vi "setPolarity.vi"(0 "SingleAxisController in":refnum<class "_SingleAxisController.lvclass">, 2 "polarity_items (in)":T2[](array[typedef]), 3 "axis (in) - nc-this is only applicable for multi-axis applications":T1, 5 "error in (no error)":errorcluster) -> (14 "SingleAxisController out":refnum<class "_SingleAxisController.lvclass">, 17 "success?":bool, 18 "response":string, 19 "error out":errorcluster)   [LabVIEW 2020, in "classes.lvlib" / "_SingleAxisController.lvclass"]
doc: "Produced By:\n\n<B>Kod Integrations, LLC</B>\n4835 Marianne Drive\nMount Airy, MD 21771\nhttp://www.kodintegrations.com\nemail: info@kodintegrations.com\nphone: (240) 687-1288"
uses:
  _SingleAxisController.lvclass
  C:/GEECS/Developers Version/source/Device Drivers/Newmark-NSC-A/Arcus Driver 3.0.0/ArcusUsbComm/classes/Controller/_Controller.lvclass
  common/controls/polarity_item.ctl
  common/controls/polarity.ctl
  common/controls/axis.ctl
  common/controls/simple_actions.ctl
  libraries/common.lvlib
  Controller/_Controller.lvclass
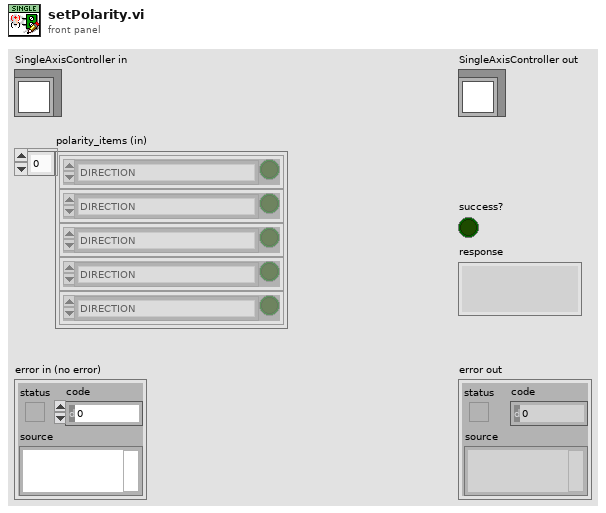
[diagram p1: front panel]
types:
  T1 = typedef "common.lvlib/axis.ctl" = enum16{"X", "Y", "Z", "U"}
  T2 = typedef "common.lvlib/polarity_item.ctl" = cluster{"item":T3, "status":bool}
  T3 = typedef "common.lvlib/polarity.ctl" = enum16{"DIRECTION", "LIMIT", "HOME", "DIG_OUT", "DIG_IN", "ENABLE_OUT", "JUMP_ERR", "LATCH", "Z-CHAN_INDEX", "ENCODER_DECODING:1X", "ENCODER_DECODING:2X", "ENCODER_DECODING:4X", "ALARM", "STANDALONE_ERR", "-", "<reserved/nc>"}
  T4 = typedef "common.lvlib/simple_actions.ctl" = enum16{"from_value", "to_value"}
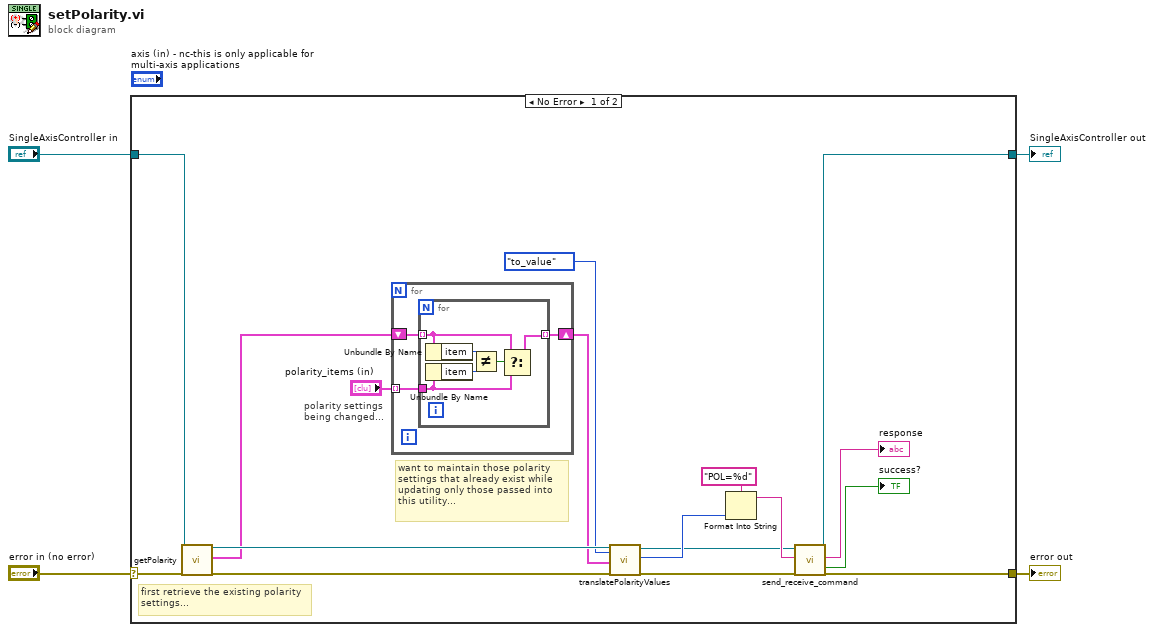
[diagram p0: block diagram]
diagram:
  n1 = case shown="No Error" "error in (no error)" {
    selector: "error in (no error)" -> [w8 w32]
    tunnel: [w7 w32] -> w3
    tunnel: [w5 w31] -> w1
    tunnel: "SingleAxisController in" -> [w6 w31]
    frame No Error {
      # "want to maintain those polarity\nsettings that already exist while\nupdating only those passed into\nthis utility..."
      # "first retrieve the existing polarity\nsettings..."
      # "polarity settings\nbeing changed..."
      n2 = call-dynamic "getPolarity.vi"("reference (in)"=w6, "error in (no error)"=w8) -> ("reference (out)"=w21:refnum<class "_SingleAxisController.lvclass">, "polarity_items (out)"=w9:T2[], "error out"=w13:errorcluster)  [unwired: 15 in]
      n3 = for {
        tunnel: "polarity_items (in)" -> [w23] mode=indexing
        shift-right: [w22] -> w11
        shift-left: w9 -> [w24]
        n4 = for {
          tunnel: w24 -> [w27] mode=indexing
          tunnel: w23 -> [w26]
          tunnel: [w25] -> w22 mode=indexing
          n5 = Unbundle By Name(w27) -> ("item"=w30:T3)
          n6 = Unbundle By Name(w26) -> ("item"=w29:T3)
          n7 = Not Equal?(x=w30, y=w29) -> (x != y?=w28:bool)
          n8 = Select(t=w27, s=w28, f=w26) -> (s? t:f=w25:T2)
        }
      }
      n9 = call-dynamic "translatePolarityValues.vi"("SingleAxisController in"=w21, "simple_actions"=simple_actions."to_value", "polarity_items (in)"=w11, "error in (no error)"=w13) -> ("SingleAxisController out"=w16:refnum<class "_SingleAxisController.lvclass">, "polarity_value (out)"=w20:u32, "error out"=w14:errorcluster)  [unwired: 12 in, 1 out]
      n10 = Format Into String(format string="POL=%d", w20) -> (resulting string=w17:string)  [unwired: 2 in, 1 out]
      n11 = call "send_receive_command.vi"("reference (in)"=w16, "ASCII Command (in)"=w17, "error in (no error)"=w14) -> ("reference (out)"=w5:refnum<class "_SingleAxisController.lvclass">, "response (out)"=→"response":string, "success?"=→"success?":bool, "error out"=w7:errorcluster)  [unwired: 12 in, 1 out]
    }
    frame Error {
    }
  }
  "error out" <- w3
  "SingleAxisController out" <- w1
